vi "Finalize To Settings.vi"(8 "error in (no error)":errorcluster, 11 "UDP Thread Configuration in":refnum<class "UDP Thread Configuration.lvclass">) -> (0 "error out":errorcluster, 2 "settings":cluster{"key":string, "value":string}[](array[cluster]), 3 "UDP Thread Configuration out":refnum<class "UDP Thread Configuration.lvclass">)   [LabVIEW 2017, in "UDP.lvlib" / "UDP Thread Configuration.lvclass"]
uses:
  UDP Thread Configuration.lvclass
  UDP Thread Configuration.lvclass/UDP Thread Configuration.ctl
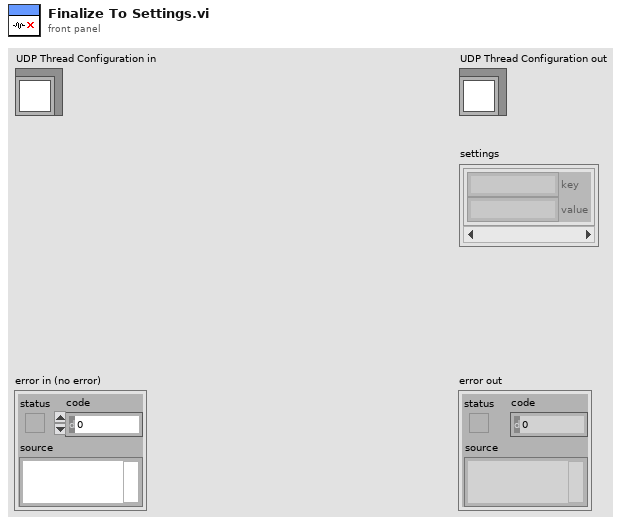
[diagram p1: front panel]
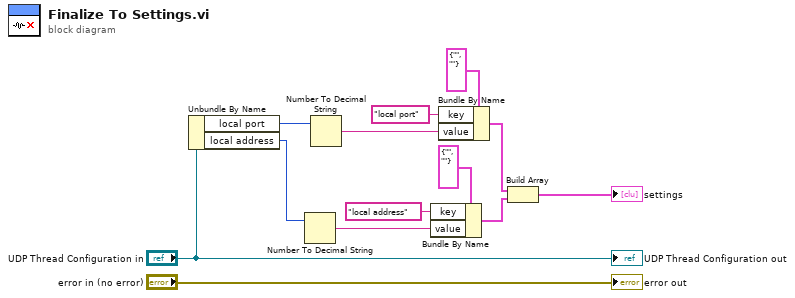
[diagram p0: block diagram]
diagram:
  n1 = Unbundle By Name("UDP Thread Configuration in") -> ("local port"=w13:u16, "local address"=w2:u32)
  n2 = Number To Decimal String(number=w2) -> (decimal integer string=w1:string)  [unwired: 1 in]
  n3 = Number To Decimal String(number=w13) -> (decimal integer string=w11:string)  [unwired: 1 in]
  n4 = Bundle By Name(cluster=cluster{"key":string, "value":string} {"key"="", "value"=""} ("setting"), "key"="local address", "value"=w1) -> (w7:cluster{"key":string, "value":string})
  n5 = Bundle By Name(cluster=cluster{"key":string, "value":string} {"key"="", "value"=""} ("setting"), "key"="local port", "value"=w11) -> (w6:cluster{"key":string, "value":string})
  n6 = Build Array(w6, w7) -> (→"settings":cluster{"key":string, "value":string}[])
  "error out" <- "error in (no error)"
  "UDP Thread Configuration out" <- "UDP Thread Configuration in"
